vi "IntegrateWaveForm.vi"(4 "First chunk?":bool, 6 "Offset duration":dbl=1.0 format="%0.2f", 7 "Offset correction":dbl, 8 "error in (no error)":errorcluster, 10 "Integrate settings":cluster{"Factor":dbl, "Output name":string}={"Factor"=1.0, "Output name"=""}, 11 "Waveform":waveform(dbl)) -> (0 "error out":errorcluster, 2 "Min max":cluster{"Max":dbl, "Min":dbl}, 3 "Integrated Waveform":waveform(dbl))   [LabVIEW 2015]
uses:
  <vilib>/Analysis/2dsp.llb/Integral Method.ctl
  <vilib>/Waveform/WDTOps.llb/WDT Get Waveform Subset DBL.vi
  <vilib>/Analysis/NI_AALPro.lvlib
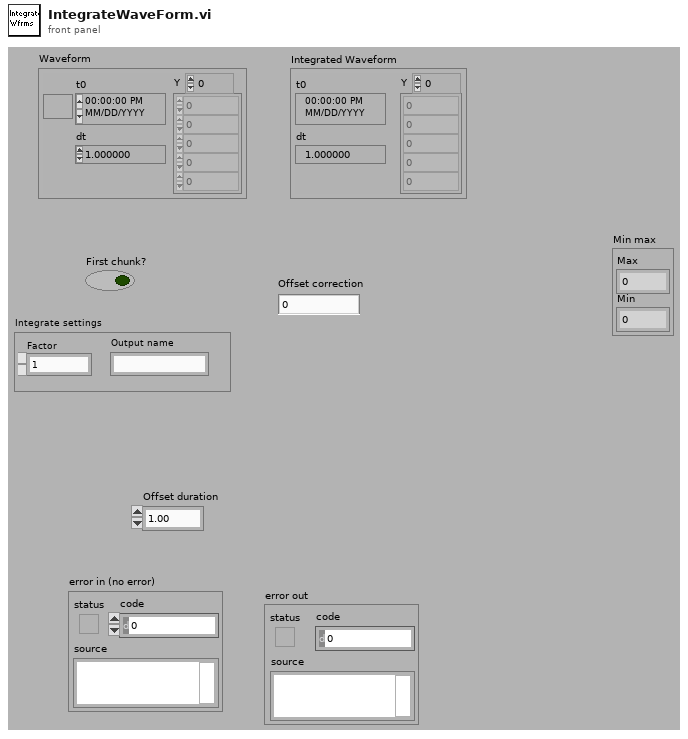
[diagram p1: front panel]
types:
  T1 = typedef "NI_AALPro.lvlib/Integral Method.ctl" = i32
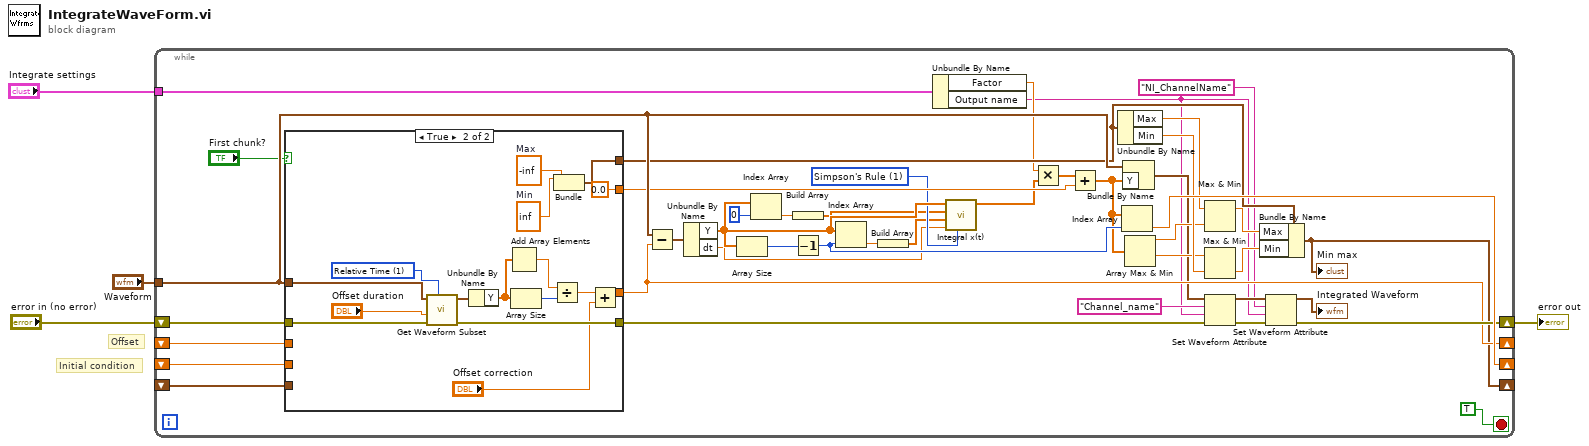
[diagram p0: block diagram]
diagram:
  # "Initial condition"
  # "Offset"
  n1 = while {
    shift-right: [w44] -> _
    shift-left: _ -> [w37]
    shift-right: [w45] -> w3
    shift-left: "error in (no error)" -> [w38]
    shift-right: [w46] -> _
    shift-left: _ -> [w36]
    tunnel: "Waveform" -> [w43]
    shift-right: [w5] -> _
    shift-left: _ -> [w41]
    tunnel: "Integrate settings" -> [w7]
    stop <- TRUE stop-if-true
    w14 = T1 1 items=["Trapezoidal Rule", "Simpson's Rule", "Simpson's 3/8 Rule", "Bode Rule"] ("integration method")
    n2 = case shown="True" "First chunk?" {
      tunnel: [w51 w53] -> w44
      tunnel: w43 -> [_ w54]
      tunnel: w37 -> [w51 _]
      tunnel: w36 -> [w50 _]
      tunnel: [w50 0.0] -> w35
      tunnel: [w48 w65] -> w39
      tunnel: [w49 w64] -> w40
      tunnel: w41 -> [w49 _]
      tunnel: w38 -> [w48 w63]
      frame False {
      }
      frame True {
        w55 = u16 1 items=["Index", "Relative Time"] ("start/duration format")
        w61 = inf  # Min
        w60 = -inf  # Max
        n3 = call-poly <vilib>:"Get Waveform Subset.vi"("start/duration format"=w55, "error in (no error)"=w63, "duration"="Offset duration", "waveform in"=w54) -> ("error out"=w65:errorcluster, "waveform out"=w59:waveform(dbl))  [unwired: 1 in, 3 out]
        n4 = Unbundle By Name(w59) -> ("Y"=w57:dbl[])
        n5 = Add Array Elements(numeric array=w57) -> (sum=w58:dbl)
        n6 = Array Size(array=w57) -> (size(s)=w56:i32)
        n7 = Divide(x=w58, y=w56) -> (x/y=w66:dbl)
        n8 = Bundle("Max"=w60, "Min"=w61) -> (w64:cluster{"Max":dbl, "Min":dbl})  [unwired: 1 out]
        n9 = Add(x=w66, y="Offset correction") -> (x+y=w53:dbl)
      }
    }
    n10 = Subtract(x=w43, y=w44) -> (x-y=w34:waveform(dbl))
    n11 = Unbundle By Name(w34) -> ("Y"=w15:dbl[], "dt"=w9:dbl)
    n12 = Array Size(array=w15) -> (size(s)=w32:i32)
    n13 = Index Array(array=w15, index=0) -> (element=w13:dbl)
    n14 = Build Array(w13) -> (w12:dbl[])
    n15 = Decrement(x=w32) -> (x-1=w31:i32)
    n16 = Index Array(array=w15, index=w31) -> (element=w11:dbl)
    n17 = Build Array(w11) -> (w10:dbl[])
    n18 = Unbundle By Name(w7) -> ("Factor"=w17:dbl, "Output name"=w16:string)
    n19 = call <vilib>:"Integral x(t).vi"("integration method"=w14, "dt"=w9, "Final Condition"=w10, "Initial Condition"=w12, "X"=w15) -> ("Integral X"=w8:dbl[])  [unwired: 5 in, 1 out]
    n20 = Multiply(x=w17, y=w8) -> (x*y=w30:dbl[])
    n21 = Add(x=w30, y=w35) -> (x+y=w29:dbl[])
    n22 = Unbundle By Name(w40) -> ("Max"=w26:dbl, "Min"=w28:dbl)
    n23 = Index Array(array=w29, index=w31) -> (element=w46:dbl)
    n24 = Bundle By Name(cluster=w43, "Y"=w29) -> (w22:waveform(dbl))
    n25 = Array Max & Min(array=w29) -> (max value=w25:dbl, min value=w27:dbl)  [unwired: 2 out]
    n26 = Max & Min(x=w26, y=w25) -> (max(x,y)=w24:dbl)  [unwired: 1 out]
    n27 = Max & Min(x=w27, y=w28) -> (min(x,y)=w23:dbl)  [unwired: 1 out]
    n28 = Set Waveform Attribute(4:w39, 5:w16, 6:"Channel_name" ("name"), 7:w22) -> (0:w19:errorcluster, 3:w21:waveform(dbl))  [unwired: 1 out]
    n29 = Bundle By Name(cluster=w40, "Max"=w24, "Min"=w23) -> (w5:cluster{"Max":dbl, "Min":dbl})
    "Min max" <- w5
    n30 = Set Waveform Attribute(4:w19, 5:w16, 6:"NI_ChannelName" ("name"), 7:w21) -> (0:w45:errorcluster, 3:→"Integrated Waveform":waveform(dbl))  [unwired: 1 out]
  }
  "error out" <- w3
